vi "FrameNo.vi"(8 "error in (no error)":errorcluster, 11 ".NET Refnum in":refnum<k24>) -> (0 "error out":errorcluster, 1 "FrameNumber":dbl format="%.2f", 3 ".NET Reference out":refnum<k24>)   [LabVIEW 2024]
uses:
  C:/Users/ROAR/Documents/Rob Motor Assessment stuff/Labview/RobUST_3D_with_Unity_Control_PXI_Low_Level_Only_Streamlined/Vicon_files/ViconDataStreamSDK_DotNET.dll
  Vicon_files/ViconDataStreamSDK_DotNET.dll
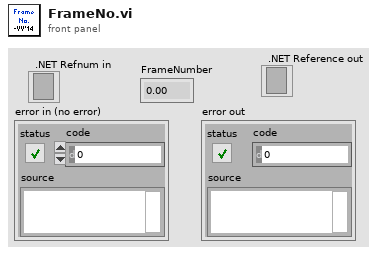
[diagram p1: front panel]
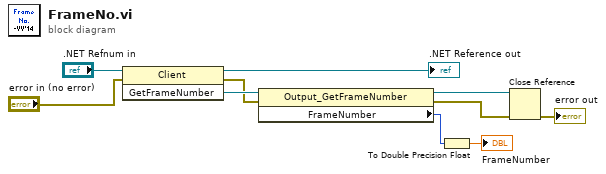
[diagram p0: block diagram]
diagram:
  n1 = invoke class="Client" method="GetFrameNumber"(reference=".NET Refnum in", error in="error in (no error)") -> (reference out=→".NET Reference out":refnum<k24>, error out=w6:errorcluster, "GetFrameNumber"=w10:refnum<k24>)  [unwired: 1 in]
  n2 = property class="Output_GetFrameNumber"(reference=w10, error in=w6) -> (reference out=w4:refnum<k24>, error out=w5:errorcluster, "FrameNumber"=w2:u32)
  n3 = To Double Precision Float(number=w2) -> (double precision float=→"FrameNumber":dbl)
  n4 = Close Reference(reference=w4, error in (no error)=w5) -> (error out=→"error out":errorcluster)
